vi "Update.vi"(8 "error in (no error)":errorcluster, 10 "Message in":refnum<class "UpdateMessage.lvclass">, 11 "DAQCascade512II in":refnum<class "DAQCascade512II.lvclass">) -> (0 "error out":errorcluster, 3 "DAQCascade512II out":refnum<class "DAQCascade512II.lvclass">)   [LabVIEW 2012, in "DAQCascade512II.lvclass"]
doc: "The update method processes the command 'update'. \n\nThe command 'update' is used for receiving new values to be set to the private data of the class. This could be seen as a public set method for setting new parameters to the private class data."
uses:
  DAQCascade512II.lvclass
  <vilib>/Distrio/Murmex/UpdateMessage/UpdateMessage.lvclass
  DAQCascade512II.lvclass/DAQCascade512II.ctl
  <vilib>/Distrio/Murmex/Murmex/Murmex.lvclass
panel:
  # "This method is called when the UPDATE\ntrigger is sent. \n\nOverride this method when your component needs to\nrespond to this trigger. \n\nCall parent for proper implementation"
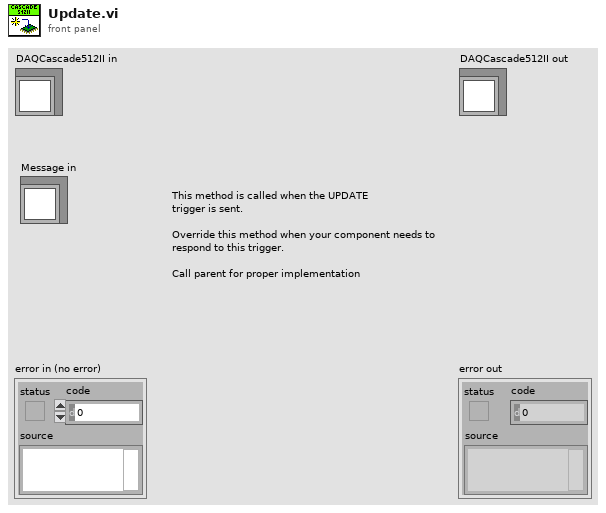
[diagram p1: front panel]
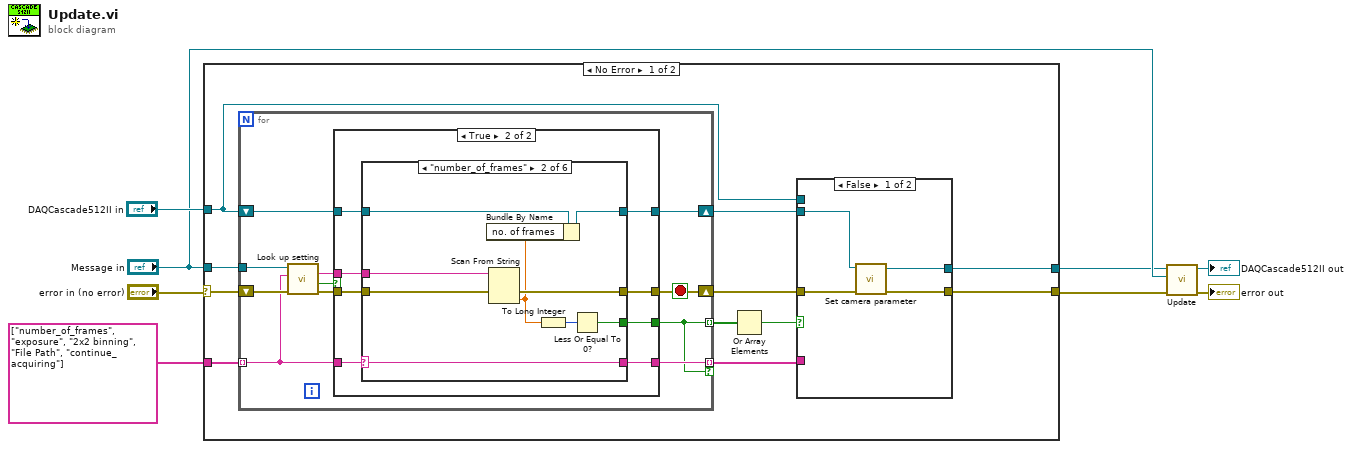
[diagram p0: block diagram]
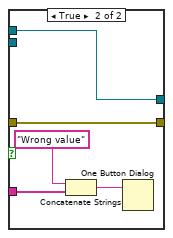
[diagram p2: hidden frame]
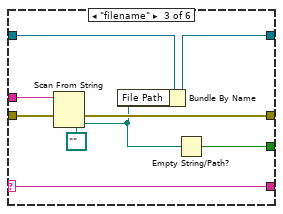
[diagram p5: hidden frame]
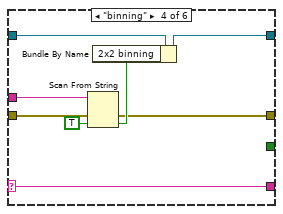
[diagram p6: hidden frame]
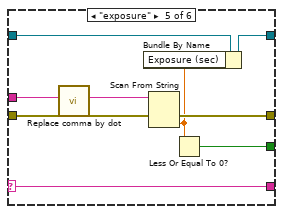
[diagram p7: hidden frame]
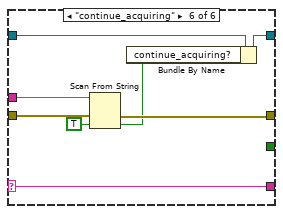
[diagram p8: hidden frame]
diagram:
  n1 = case shown="No Error" "error in (no error)" {
    selector: "error in (no error)" -> [w18 w98]
    tunnel: [w10 w98] -> w2
    tunnel: [w12 w97] -> w3
    tunnel: "Message in" -> [w19 _]
    tunnel: string[] ["number_of_frames", "exposure", "2x2 binning", "File Path", "continue_acquiring"] -> [w17 _]
    tunnel: "DAQCascade512II in" -> [w16 w97]
    frame No Error {
      n2 = for {
        tunnel: w19 -> [w38]
        shift-right: [w30] -> w9
        shift-left: w18 -> [w37]
        tunnel: w17 -> [w35] mode=indexing
        shift-right: [w33] -> w15
        shift-left: w16 -> [w34]
        tunnel: [w31] -> w11 mode=indexing if=w29
        tunnel: [w29] -> w13 mode=indexing
        stop <- w30 stop-if-true
        n3 = call <vilib>:"Look up setting.vi"("error in (no error)"=w37, "tag name"=w35, "UpdateMessage in"=w38) -> ("error out"=w36:errorcluster, "found?"=w39:bool, "value"=w32:string)  [unwired: 5 in, 1 out]
        n4 = case shown="True" w39 {
          tunnel: w36 -> [w42 w50]
          tunnel: [w42 w43] -> w30
          tunnel: w35 -> [w40 w49]
          tunnel: w34 -> [w41 w48]
          tunnel: [w41 w47] -> w33
          tunnel: w32 -> [_ w46]
          tunnel: [w40 w45] -> w31
          tunnel: [_ w44] -> w29
          frame False {
          }
          frame True {
            n5 = case shown="\"number_of_frames\"" w49 {
              selector: w49 -> [w51 w57 w71 w76 w81 w92]
              tunnel: [w53 w59 w64 w72 w85 w93] -> w43
              tunnel: w50 -> [w53 w60 w65 w77 w86 w94]
              tunnel: [w52 w61 w68 w73 w87 w90] -> w47
              tunnel: w48 -> [w52 w62 w70 w79 w88 w91]
              tunnel: w46 -> [_ w58 w67 w78 w84 w95]
              tunnel: [w51 w57 w71 w76 w81 w92] -> w45
              tunnel: [_ w56 w69 _ w80 _] -> w44
              frame Default {
              }
              frame "number_of_frames" {
                n6 = Scan From String(input string=w58, error in=w60) -> (error out=w59:errorcluster, output 1=w55:dbl)  [unwired: 3 in, 2 out]
                n7 = Bundle By Name(cluster=w62, "no. of frames"=w55) -> (w61:refnum<class "DAQCascade512II.lvclass">)
                n8 = To Long Integer(number=w55) -> (32bit integer=w54:i32)
                n9 = Less Or Equal To 0?(x=w54) -> (x <= 0?=w56:bool)
              }
              frame "filename" {
                n10 = Scan From String(input string=w67, error in=w65, default 1=path "" ("File Path")) -> (error out=w64:errorcluster, output 1=w63:path)  [unwired: 2 in, 2 out]
                n11 = Bundle By Name(cluster=w70, "File Path"=w63) -> (w68:refnum<class "DAQCascade512II.lvclass">)
                n12 = Empty String/Path?(string/path=w63) -> (empty?=w69:bool)
              }
              frame "binning" {
                n13 = Scan From String(input string=w78, error in=w77, default 1=TRUE) -> (error out=w72:errorcluster, output 1=w74:bool)  [unwired: 2 in, 2 out]
                n14 = Bundle By Name(cluster=w79, "2x2 binning"=w74) -> (w73:refnum<class "DAQCascade512II.lvclass">)
              }
              frame "exposure" {
                n15 = call <vilib>:"Replace comma by dot.vi"("input string"=w84) -> ("result string"=w83:string)  [unwired: 10 in]
                n16 = Scan From String(input string=w83, error in=w86) -> (error out=w85:errorcluster, output 1=w82:dbl)  [unwired: 3 in, 2 out]
                n17 = Bundle By Name(cluster=w88, "Exposure (sec)"=w82) -> (w87:refnum<class "DAQCascade512II.lvclass">)
                n18 = Less Or Equal To 0?(x=w82) -> (x <= 0?=w80:bool)
              }
              frame "continue_acquiring" {
                n19 = Scan From String(input string=w95, error in=w94, default 1=TRUE) -> (error out=w93:errorcluster, output 1=w89:bool)  [unwired: 2 in, 2 out]
                n20 = Bundle By Name(cluster=w91, "continue_acquiring?"=w89) -> (w90:refnum<class "DAQCascade512II.lvclass">)
              }
            }
          }
        }
      }
      n21 = Or Array Elements(Boolean array=w13) -> (logical OR=w14:bool)
      n22 = case shown="False" w14 {
        tunnel: w16 -> [_ w28]
        tunnel: w15 -> [w21 _]
        tunnel: w11 -> [_ w27]
        tunnel: [w20 w28] -> w12
        tunnel: [w22 w24] -> w10
        tunnel: w9 -> [w23 w24]
        frame False {
          n23 = call-dynamic "Set camera parameter.vi"("error in (no error)"=w23, "DAQCascade512II in"=w21) -> ("error out"=w22:errorcluster, "DAQCascade512II out"=w20:refnum<class "DAQCascade512II.lvclass">)  [unwired: 8 in]
        }
        frame True {
          n24 = Concatenate Strings("Wrong value" ("string"), w27) -> (w26:string)
          n25 = One Button Dialog(message=w26) -> ()  [unwired: 1 in, 1 out]
        }
      }
    }
    frame Error {
    }
  }
  n26 = call-parent "Update.vi"("error in (no error)"=w2, "Message in"="Message in", "Murmex in"=w3) -> ("error out"=→"error out":errorcluster, "Murmex out"=→"DAQCascade512II out":refnum<class "DAQCascade512II.lvclass">)  [unwired: 7 in]
